vi "testJobber.vi"(8 "error in (no error)":errorcluster, 11 "TestCase in":refnum<class "Test Jobber.lvclass">) -> (0 "error out":errorcluster, 3 "TestCase out":refnum<class "Test Jobber.lvclass">)   [LabVIEW 2014, in "Test Jobber.lvclass"]
uses:
  Test Jobber.lvclass
  <vilib>/addons/_JKI Toolkits/VI Tester/TestCase.llb/TestCase.lvclass
  Core/LabVIEW CI Service/Actors/Jobber/Jobber/Jobber.lvclass
  Jobber Test Code/Dummy Job/Dummy Job.lvclass
  Core/LabVIEW CI Service/Classes/Job/Job.lvclass
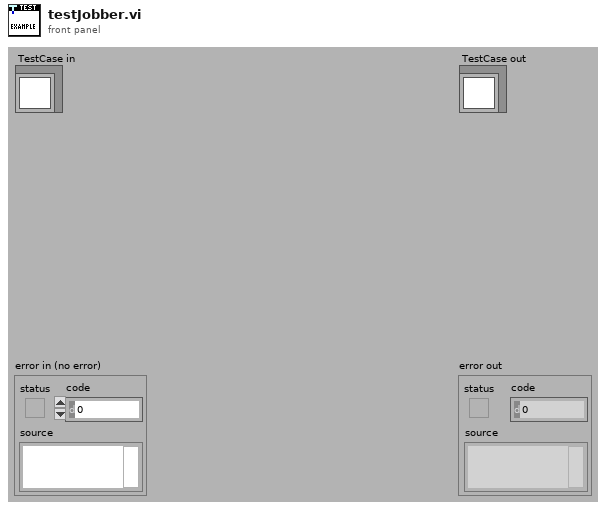
[diagram p1: front panel]
types:
  T1 = typedef "Job Results - STYP.ctl" = cluster{"Status":u16, "Text":string, "Executor Number":i32}
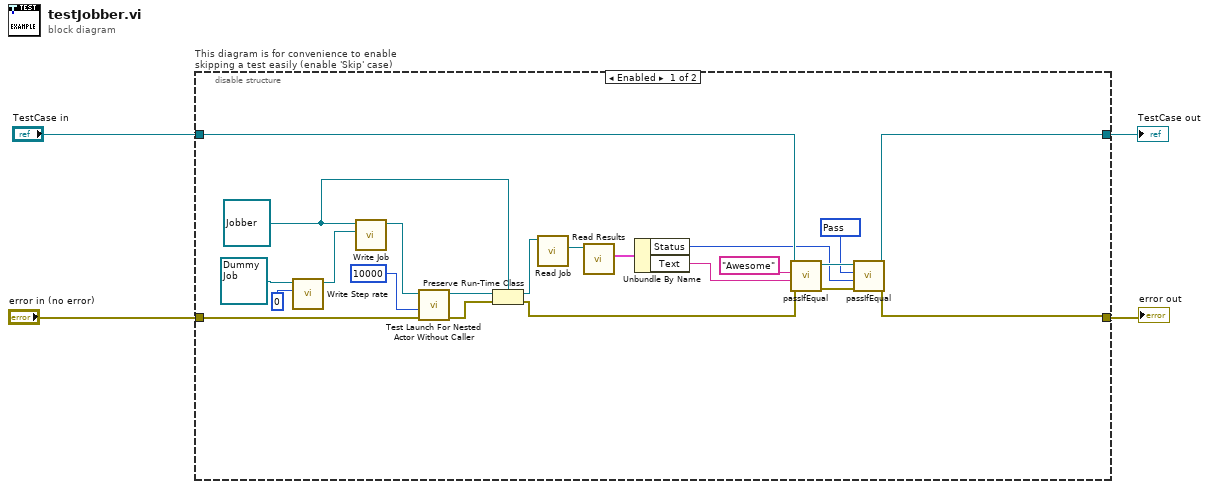
[diagram p0: block diagram]
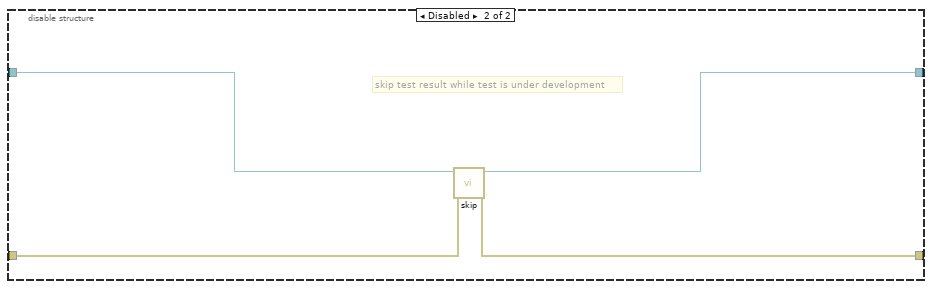
[diagram p2: hidden frame]
diagram:
  n1 = disable-structure "This diagram is for convenience to enable skipping a test easily (enable 'Skip' case)" shown="Enabled" {
    disable-tunnel: "TestCase in" -> [w16 w30]
    disable-tunnel: [w26 w28] -> w1
    disable-tunnel: [w8 w29] -> w3
    disable-tunnel: "error in (no error)" -> [w23 w27]
    frame Enabled {
      w10 = u16 200 items=["Service Error"=504, "Abort"=503, "Fail"=500, "Pass"=200] ("Status")
      w21 = refnum<class "Jobber.lvclass"> refnum ("Jobber.lvlib:Jobber.lvclass")
      n2 = call "Write Step rate.vi"("Step rate"=u32 0, "Dummy Job in"=refnum<class "Dummy Job.lvclass"> refnum ("Dummy Job.lvclass")) -> ("Dummy Job out"=w6:refnum<class "Dummy Job.lvclass">)  [unwired: 9 in]
      n3 = call "Write Job.vi"("Job.lvclass"=w6, "Jobber in"=w21) -> ("Jobber out"=w24:refnum<class "Jobber.lvclass">)  [unwired: 9 in]
      n4 = call "Test Launch For Nested Actor Without Caller.vi"("error in (no error)"=w23, "timeout in ms (-1)"=10000, "Actor Before Launch"=w24) -> ("error out"=w19:errorcluster, "Actor After Stop"=w22:refnum<class "Actor.lvclass">)  [unwired: 7 in]
      n5 = Preserve Run-Time Class(object in=w22, error in=w19, 2:w21) -> (object out=w20:refnum<class "Jobber.lvclass">, error out=w9:errorcluster)
      n6 = call "Read Job.vi"("Jobber in"=w20) -> ("Job.lvclass"=w18:refnum<class "Job.lvclass">)  [unwired: 10 in]
      n7 = call "Read Results.vi"("Job in"=w18) -> ("Results"=w14:T1)  [unwired: 10 in]
      n8 = Unbundle By Name(w14) -> ("Status"=w11:u16, "Text"=w13:string)
      n9 = call-dynamic "passIfEqual.vi"("error in (no error)"=w9, "y"=w13, "x"="Awesome" ("Text"), "TestCase in"=w16) -> ("error out"=w17:errorcluster, "TestCase out"=w15:refnum<class "Test Jobber.lvclass">)  [unwired: 6 in]
      n10 = call-dynamic "passIfEqual.vi"("error in (no error)"=w17, "y"=w11, "x"=w10, "TestCase in"=w15) -> ("error out"=w8:errorcluster, "TestCase out"=w26:refnum<class "Test Jobber.lvclass">)  [unwired: 6 in]
    }
    frame Disabled {
      # "skip test result while test is under development"
      n11 = call <vilib>:"skip.vi"("error in (no error)"=w27, "TestCase in"=w30) -> ("error out"=w29:errorcluster, "TestCase out"=w28:refnum<class "Test Jobber.lvclass">)  [unwired: 8 in]
    }
  }
  "error out" <- w3
  "TestCase out" <- w1
